vi "로봇1.vi"() -> ()   [LabVIEW 2015]
uses:
  <vilib>/NXT/Block Support/NXT_InputPort.ctl
  <vilib>/NXT/Block Support/NXT_OutputPort.ctl
  <vilib>/NXT/Dual Mode Library/Sensors/Sonar_cm.vi
  <vilib>/NXT/Dual Mode Library/Sensors/Light_On.vi
  <vilib>/NXT/NXTIO Xnodes/NXTIONodeSubVIs/NXTMoveMotors.vi
  <vilib>/NXT/Dual Mode Library/Waits/Wait_Num.vi
  <vilib>/NXT/Dual Mode Library/Waits/Wait_Rotation.vi
  <vilib>/NXT/NXTIO Xnodes/AddressXNode/NXTIOAddress.xnode
  <vilib>/NXT/Subs/LVHSConnector.ctl
  <vilib>/NXT/NXTIO Xnodes/NXTIOXNode/NXTIO.xnode
  <vilib>/NXT/LegoClasses/BrickReference/BrickReference.lvclass
panel:
  in  "stop":bool
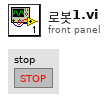
[diagram p1: front panel]
types:
  T1 = typedef "NXT_InputPort.ctl" = u32
  T2 = typedef "NXT_OutputPort.ctl" = u8
  T3 = typedef "LVHSConnector.ctl" = refnum<class "BrickReference.lvclass">
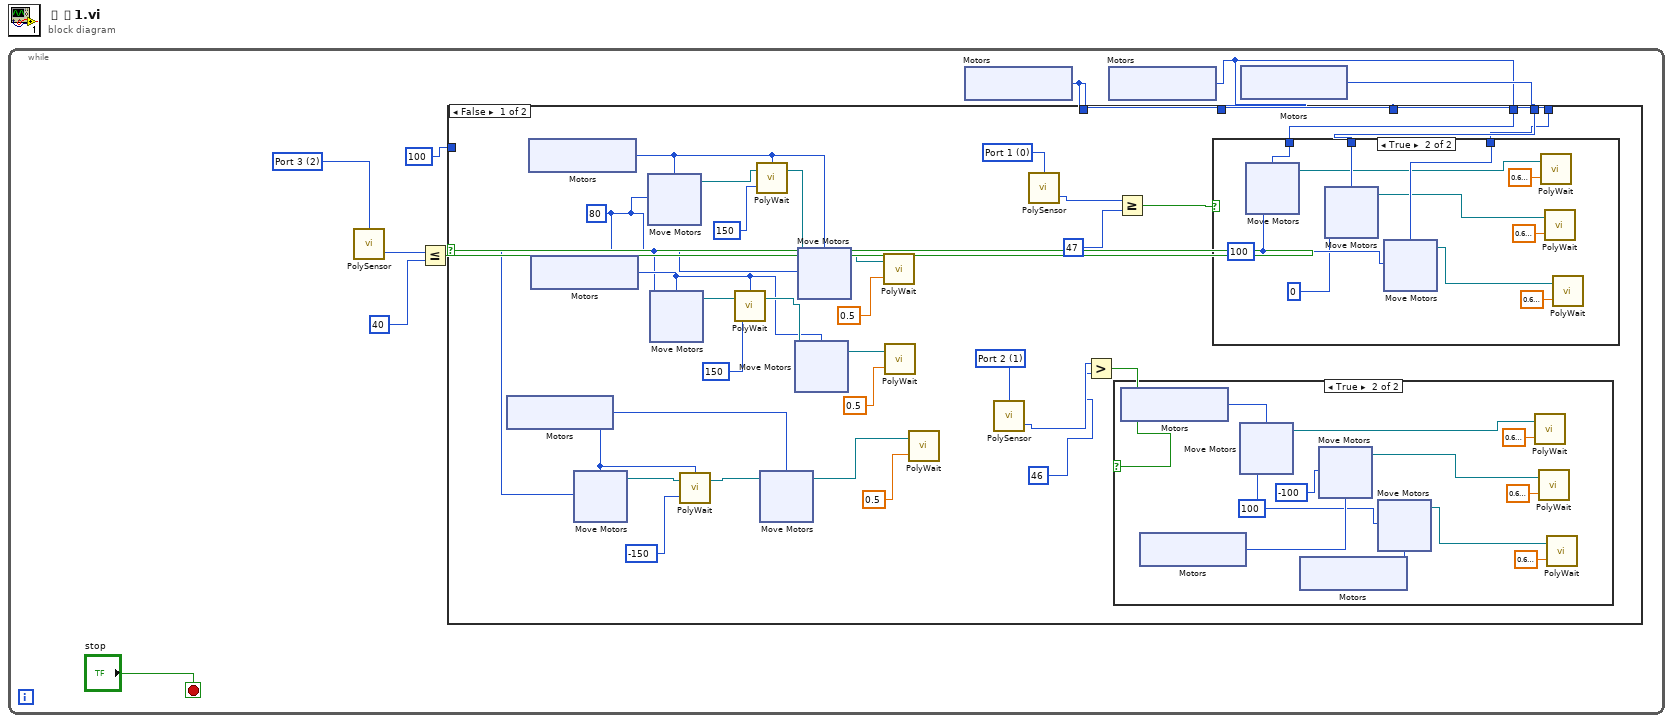
[diagram p0: block diagram]
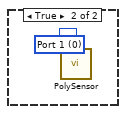
[diagram p4: hidden frame]
diagram:
  n1 = while {
    stop <- "stop" stop-if-true
    w9 = T1 2 items=["Port 1", "Port 2", "Port 3", "Port 4"] ("Port (Port 4)")
    n2 = call-poly <vilib>:"PolySensor.vi"("Port (Port 4)"=w9) -> ("Distance (cm)"=w5:i16)  [unwired: 2 in, 1 out]
    n3 = Less Or Equal?(x=w5, y=i16 40) -> (x <= y?=w7:bool)
    n4 = xnode "Motors"() -> ("Motor"=w2:T2)
    n5 = xnode "Motors"() -> ("Motor"=w3:T2)
    n6 = xnode "Motors"() -> ("Motor"=w4:T2)
    n7 = case shown="False" w7 {
      tunnel: w2 -> [w37 _]
      tunnel: w3 -> [w39 _]
      tunnel: w4 -> [w38 _]
      tunnel: w2 -> [_ _]
      tunnel: w3 -> [_ _]
      tunnel: w2 -> [_ _]
      tunnel: i8 100 ("Power/Speed 1") -> [_ _]
      frame False {
        w13 = i8 80 ("Power/Speed 1")
        w32 = T1 1 items=["Port 1", "Port 2", "Port 3", "Port 4"] ("Port (Port 3)")
        w33 = T1 0 items=["Port 1", "Port 2", "Port 3", "Port 4"] ("Port (Port 3)")
        n8 = xnode "Motors"() -> ("Motor"=w20:T2)
        n9 = xnode "Motors"() -> ("Motor"=w27:T2)
        n10 = xnode "Motors"() -> ("Motor"=w14:T2)
        n11 = xnode "Move Motors"("Power/Speed 1"=w13, "Motors"=w20) -> ("NXT/EV3"=w25:T3)  [unwired: 1 in]
        n12 = xnode "Move Motors"("Power/Speed 1"=w13, "Motors"=w27) -> ("NXT/EV3"=w31:T3)  [unwired: 1 in]
        n13 = xnode "Move Motors"("Power/Speed 1"=w13, "Motors"=w14) -> ("NXT/EV3"=w16:T3)  [unwired: 1 in]
        n14 = call-poly <vilib>:"PolyWait.vi"("Position Change (180)"=-150, "NXT/EV3"=w25, "Port (Port A)"=w20) -> ("NXT/EV3"=w24:T3)  [unwired: 1 in]
        n15 = call-poly <vilib>:"PolyWait.vi"("Position Change (180)"=150, "NXT/EV3"=w16, "Port (Port A)"=w14) -> ("NXT/EV3"=w17:T3)  [unwired: 1 in]
        n16 = call-poly <vilib>:"PolyWait.vi"("Position Change (180)"=150, "NXT/EV3"=w31, "Port (Port A)"=w27) -> ("NXT/EV3"=w30:T3)  [unwired: 1 in]
        n17 = xnode "Move Motors"("Motors"=w20, "NXT/EV3"=w24) -> ("NXT/EV3"=w23:T3)  [unwired: 1 in]
        n18 = xnode "Move Motors"("Motors"=w14, "NXT/EV3"=w17) -> ("NXT/EV3"=w18:T3)  [unwired: 1 in]
        n19 = xnode "Move Motors"("Power/Speed 1"=w13, "Motors"=w27, "NXT/EV3"=w30) -> ("NXT/EV3"=w29:T3)
        n20 = call-poly <vilib>:"PolyWait.vi"("Time (1 sec)"=sgl 0.5, "NXT/EV3"=w29) -> ()  [unwired: 2 in, 1 out]
        n21 = call-poly <vilib>:"PolyWait.vi"("Time (1 sec)"=sgl 0.5, "NXT/EV3"=w18) -> ()  [unwired: 2 in, 1 out]
        n22 = call-poly <vilib>:"PolyWait.vi"("Time (1 sec)"=sgl 0.5, "NXT/EV3"=w23) -> ()  [unwired: 2 in, 1 out]
        n23 = call-poly <vilib>:"PolySensor.vi"("Port (Port 3)"=w32) -> ("Scaled Value"=w36:i16)  [unwired: 2 in, 1 out]
        n24 = call-poly <vilib>:"PolySensor.vi"("Port (Port 3)"=w33) -> ("Scaled Value"=w42:i16)  [unwired: 2 in, 1 out]
        n25 = Greater?(x=w36, y=i16 46) -> (0:w34:bool)
        n26 = case shown="True" w34 {
          frame False {
          }
          frame True {
            w89 = i8 100 ("Power/Speed 1")
            n27 = xnode "Motors"() -> ("Motor"=w92:T2)
            n28 = xnode "Motors"() -> ("Motor"=w91:T2)
            n29 = xnode "Move Motors"("Power/Speed 1"=w89, "Motors"=w92) -> ("NXT/EV3"=w95:T3)  [unwired: 1 in]
            n30 = xnode "Motors"() -> ("Motor"=w90:T2)
            n31 = xnode "Move Motors"("Power/Speed 1"=i8 -100, "Motors"=w91) -> ("NXT/EV3"=w94:T3)  [unwired: 1 in]
            n32 = xnode "Move Motors"("Power/Speed 1"=w89, "Motors"=w90) -> ("NXT/EV3"=w93:T3)  [unwired: 1 in]
            n33 = call-poly <vilib>:"PolyWait.vi"("Time (1 sec)"=sgl 0.7, "NXT/EV3"=w95) -> ()  [unwired: 2 in, 1 out]
            n34 = call-poly <vilib>:"PolyWait.vi"("Time (1 sec)"=sgl 0.7, "NXT/EV3"=w94) -> ()  [unwired: 2 in, 1 out]
            n35 = call-poly <vilib>:"PolyWait.vi"("Time (1 sec)"=sgl 0.7, "NXT/EV3"=w93) -> ()  [unwired: 2 in, 1 out]
          }
        }
        n36 = Greater Or Equal?(x=w42, y=i16 47) -> (x >= y?=w40:bool)
        n37 = case shown="True" w40 {
          tunnel: w39 -> [_ w133]
          tunnel: w38 -> [_ w132]
          tunnel: w37 -> [_ w131]
          frame False {
          }
          frame True {
            w124 = i8 100 ("Power/Speed 1")
            n38 = xnode "Move Motors"("Power/Speed 1"=w124, "Motors"=w133) -> ("NXT/EV3"=w127:T3)  [unwired: 1 in]
            n39 = xnode "Move Motors"("Power/Speed 1"=i8 0, "Motors"=w132) -> ("NXT/EV3"=w126:T3)  [unwired: 1 in]
            n40 = xnode "Move Motors"("Power/Speed 1"=w124, "Motors"=w131) -> ("NXT/EV3"=w125:T3)  [unwired: 1 in]
            n41 = call-poly <vilib>:"PolyWait.vi"("Time (1 sec)"=sgl 0.7, "NXT/EV3"=w127) -> ()  [unwired: 2 in, 1 out]
            n42 = call-poly <vilib>:"PolyWait.vi"("Time (1 sec)"=sgl 0.7, "NXT/EV3"=w126) -> ()  [unwired: 2 in, 1 out]
            n43 = call-poly <vilib>:"PolyWait.vi"("Time (1 sec)"=sgl 0.7, "NXT/EV3"=w125) -> ()  [unwired: 2 in, 1 out]
          }
        }
      }
      frame True {
        w155 = T1 0 items=["Port 1", "Port 2", "Port 3", "Port 4"] ("Port (Port 3)")
        n44 = call-poly <vilib>:"PolySensor.vi"("Port (Port 3)"=w155) -> ()  [unwired: 2 in, 2 out]
      }
    }
  }
